vi "DataLogger.contents.vi"   [LabVIEW 2014, in "DataLogger.lvlib"]
uses:
  DataLogger.lvlib
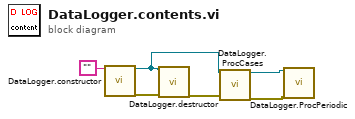
[diagram p0: block diagram]
diagram:
  n1 = call "DataLogger.constructor.vi"("name"="") -> ("i ref out"=w6:refnum<vi>, "error out"=w3:errorcluster)  [unwired: 16 in, 1 out]
  n2 = call "DataLogger.destructor.vi"("i ref in"=w6, "error in (no error)"=w3) -> ("error out"=w2:errorcluster)  [unwired: 17 in]
  n3 = call "DataLogger.ProcCases.vi"("i ref in"=w6, "error in (no error)"=w2) -> ("i ref out"=w5:refnum<vi>, "error out"=w1:errorcluster)  [unwired: 15 in, 1 out]
  n4 = call "DataLogger.ProcPeriodic.vi"("i ref in"=w5, "error in (no error)"=w1) -> ()  [unwired: 15 in, 3 out]
